vi "Shutter Mode.vi"(0 "Notifier Name":string, 7 "Progressive Mode?":bool, 11 "Error In":errorcluster) -> (4 "Notifier Name DUP":string, 15 "Error Out":errorcluster)   [LabVIEW 2020]
uses:
  Hardware Configuration/Hardware Configuration Controls/Company.ctl
  Hamamatsu/Orca Flash/Orca Flash Controls/Orca Flash Actions.ctl
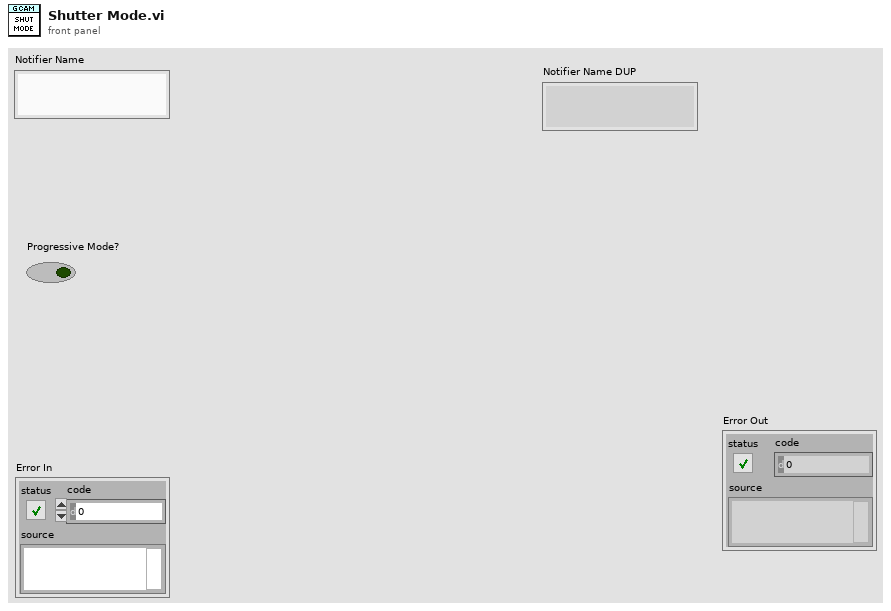
[diagram p1: front panel]
types:
  T1 = typedef "Company.ctl" = enum16{"AA Opto Electronic", "ASI", "Coherent", "CVI", "DAQmx", "Hamamatsu", "IDS", "Mad City Labs", "Marzhauser", "Measurement Computing", "MPB Com", "Photometrics", "PI", "Prior", "Thorlabs"}
  T2 = typedef "Orca Flash Actions.ctl" = enum16{"IDLE", "PREVIEW", "RECORD", "Record Settings", "SETPARAM", "GETPARAM", "SETROI", "GETROI", "PROGRESSIVE MODE", "AREA MODE", "STATUS", "QUIT"}
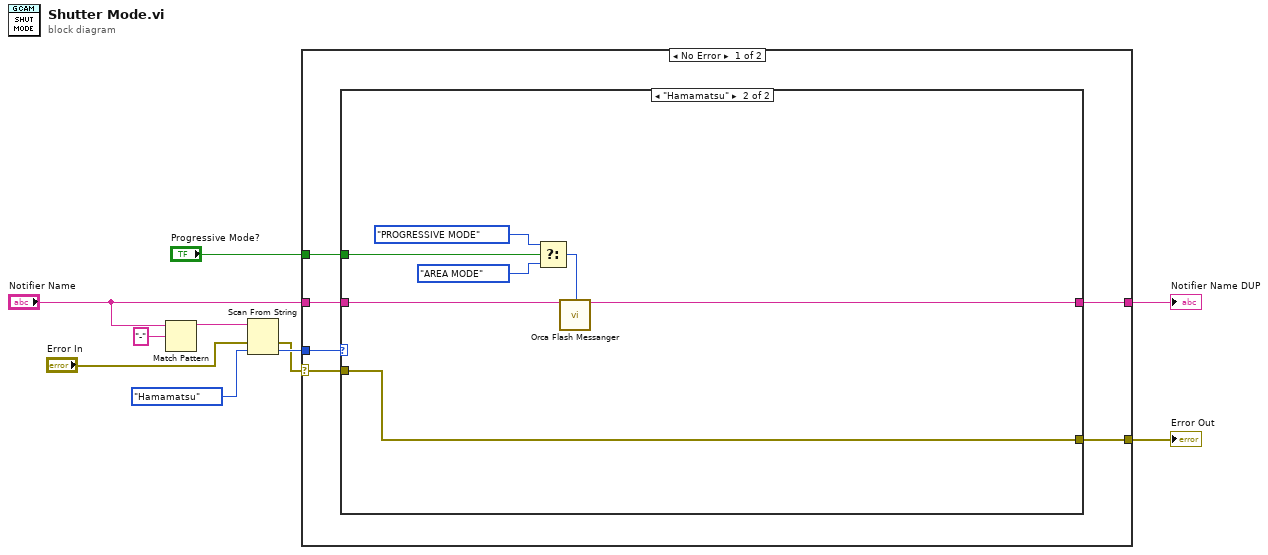
[diagram p0: block diagram]
diagram:
  n1 = Match Pattern(string="Notifier Name", regular expression="-") -> (before substring=w8:string)  [unwired: 1 in, 3 out]
  n2 = Scan From String(input string=w8, error in="Error In", default 1=Company."Hamamatsu" ("Company")) -> (error out=w4:errorcluster, output 1=w7:T1)  [unwired: 2 in, 2 out]
  n3 = case shown="No Error" w4 {
    selector: w4 -> [w14 w26]
    tunnel: w7 -> [w16 _]
    tunnel: "Notifier Name" -> [w15 w27]
    tunnel: [w13 w27] -> w3
    tunnel: [w12 w26] -> w2
    tunnel: "Progressive Mode?" -> [w11 _]
    frame No Error {
      n4 = case shown="\"Hamamatsu\"" w16 {
        tunnel: w15 -> [w18 w25]
        tunnel: w14 -> [w17 w23]
        tunnel: [w18 w24] -> w13
        tunnel: [w17 w23] -> w12
        tunnel: w11 -> [_ w19]
        frame Default {
        }
        frame "Hamamatsu" {
          n5 = Select(t=Orca_Flash_Actions."PROGRESSIVE MODE" ("Camera Actions"), s=w19, f=Orca_Flash_Actions."AREA MODE" ("Camera Actions")) -> (s? t:f=w20:T2)
          n6 = call "Orca Flash Messanger.vi"("Notifier Name"=w25, "Camera Actions"=w20) -> ("Notifier Name Dup"=w24:string)  [unwired: 9 in, 4 out]
        }
      }
    }
    frame Error {
    }
  }
  "Error Out" <- w2
  "Notifier Name DUP" <- w3
